vi "Get Desired Size.vi"(8 "error in (no error)":errorcluster, 11 "Battery Stack in":refnum<class "Battery Stack.lvclass">) -> (0 "error out":errorcluster, 2 "Desired Size":T1, 3 "Battery Stack out":refnum<class "Battery Stack.lvclass">)   [LabVIEW 2020, in "Battery Stack.lvclass"]
uses:
  Battery Stack.lvclass
  lv-oopanel/OOPanel/ArrayPanel/Desired Size.ctl
  lv-oopanel/OOPanel/ArrayPanel/ArrayPanel.lvclass
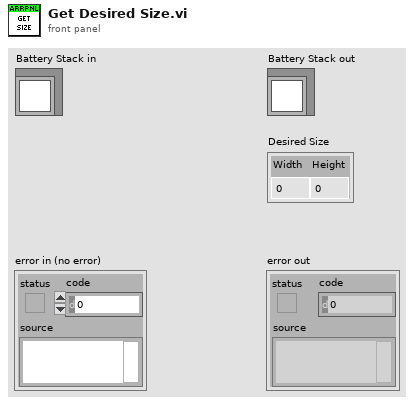
[diagram p1: front panel]
types:
  T1 = typedef "OOPanel.lvlib/ArrayPanel.lvclass/Desired Size.ctl" = cluster{"Width":u32, "Height":u32}
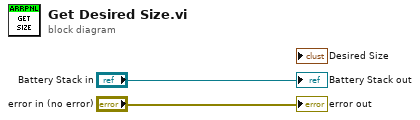
[diagram p0: block diagram]
diagram:
  "error out" <- "error in (no error)"
  "Battery Stack out" <- "Battery Stack in"
